vi "Move Channel in Wfm Grp.vi"(7 "Channels Ctrl Ref":refnum<vi>, 8 "error in (no error)":errorcluster, 10 "Before Move Index":i32, 11 "To Save Wfm Arrays":waveform(dbl)[](array[waveform])) -> (0 "error out":errorcluster, 3 "Wfm Grp Data":T1)   [LabVIEW 2025, in "TDMS Waveform Creator UI.lvlib"]
uses:
  TDMS Waveform Creator UI.lvlib
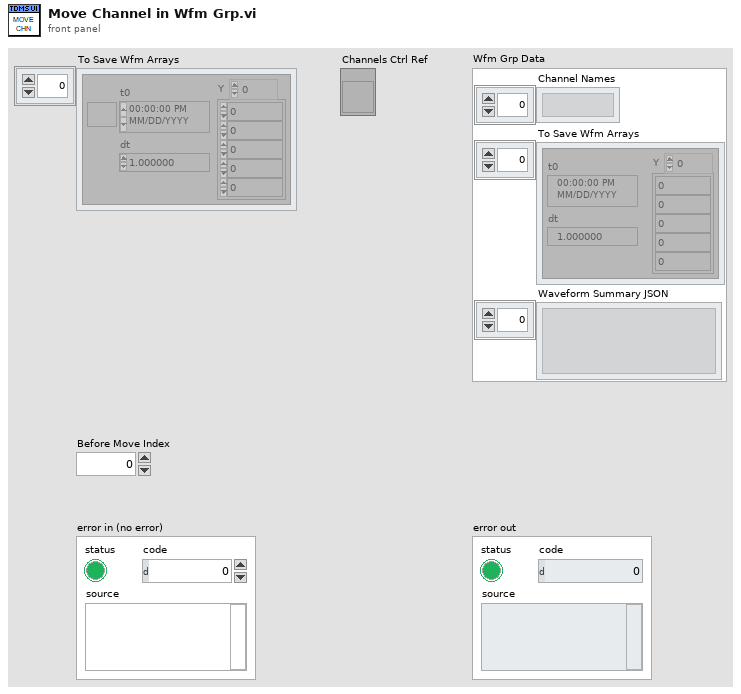
[diagram p1: front panel]
types:
  T1 = cluster{"Channel Names":string[], "To Save Wfm Arrays":waveform(dbl)[], "Waveform Summary JSON":string[]}
  T2 = cluster{"Item Names":string[], waveform(dbl)[], string[]}
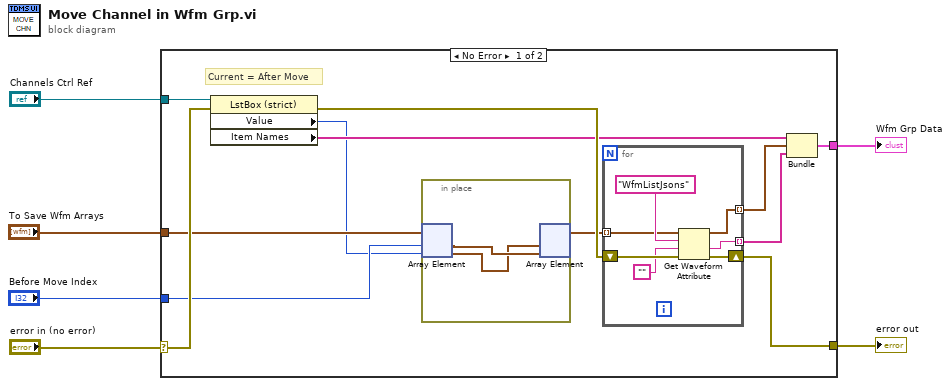
[diagram p0: block diagram]
diagram:
  n1 = case shown="No Error" "error in (no error)" {
    selector: "error in (no error)" -> [w17 w28]
    tunnel: "Channels Ctrl Ref" -> [w18 _]
    tunnel: "To Save Wfm Arrays" -> [w10 _]
    tunnel: [w15 w28] -> w3
    tunnel: [w12 _] -> w2
    tunnel: "Before Move Index" -> [w9 _]
    frame No Error {
      # "Current = After Move"
      n2 = property class="LstBox (strict)"(reference=w18, error in=w17) -> (error out=w16:errorcluster, "Value"=w8:i32, "Item Names"=w11:string[])  [unwired: 1 out]
      n3 = in-place {
        n4 = in-place-array #1(w10, w9, w8) -> (w27:waveform(dbl), w26:waveform(dbl))
        n5 = in-place-array #1(w26, w27) -> (w7:waveform(dbl)[])  [unwired: 2 out]
      }
      n6 = for {
        shift-right: [w24] -> w15
        shift-left: w16 -> [w25]
        tunnel: [w23] -> w14 mode=indexing
        tunnel: [w20] -> w13 mode=indexing
        tunnel: w7 -> [w19] mode=indexing
        n7 = Get Waveform Attribute(4:w25, 5:"", 6:"WfmListJsons" ("name"), 7:w19) -> (0:w24:errorcluster, 1:w20:string, 3:w23:waveform(dbl))  [unwired: 1 out]
      }
      n8 = Bundle("Item Names"=w11, w14, w13) -> (w12:T2)  [unwired: 1 in]
    }
    frame Error {
    }
  }
  "error out" <- w3
  "Wfm Grp Data" <- w2
